vi "Get Motor by Label.vi"(8 "error in (no error)":errorcluster, 10 "label":string, 11 "MotionSystem in":refnum<class "MotionSystem.lvclass">) -> (0 "error out":errorcluster, 1 "found":bool, 2 "Motor obj":refnum<class "Motor.lvclass">, 3 "MotionSystem out":refnum<class "MotionSystem.lvclass">)   [LabVIEW 2016, in "MotionSystem.lvlib" / "MotionSystem.lvclass"]
uses:
  <userlib>/Common Components/Hardware/Abstract System/MotionSystem/MotionSystem/MotionSystem.lvclass
  <userlib>/Common Components/Hardware/Motor/Motor/Motor.lvclass
  <userlib>/Common Components/Hardware/Abstract System/MotionSystem/MotionSystem/MotionSystem.lvclass/MotionSystem.ctl
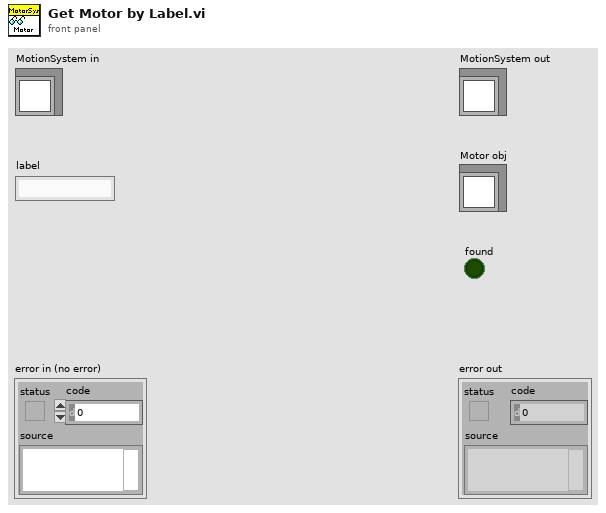
[diagram p1: front panel]
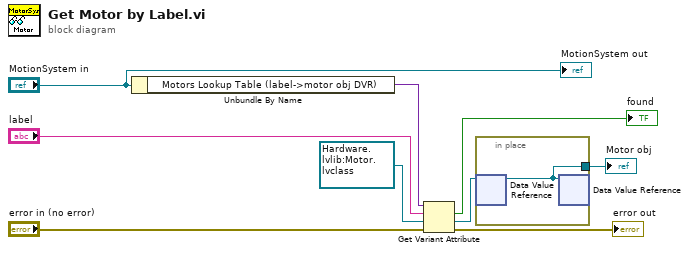
[diagram p0: block diagram]
diagram:
  n1 = Unbundle By Name("MotionSystem in") -> ("Motors Lookup Table (label->motor obj DVR)"=w8:variant)
  n2 = Get Variant Attribute(Variant=w8, name="label", default value (empty Variant)=refnum<data-value> refnum ("data value reference"), error in="error in (no error)") -> (found=→"found":bool, value=w3:refnum<data-value>, error out=→"error out":errorcluster)  [unwired: 1 out]
  n3 = in-place {
    in-place-border: [w10] -> w2
    n4 = in-place-dvr #1(w3) -> (w10:refnum<class "Motor.lvclass">)  [unwired: 1 out]
    n5 = in-place-dvr #1(w10) -> ()  [unwired: 2 out]
  }
  "Motor obj" <- w2
  "MotionSystem out" <- "MotionSystem in"
